vi "Log The Message.vi"(11 "Circle Message":refnum<class "Circle Message.lvclass">) -> (2 "log text":string="Draw Circle")   [LabVIEW 2019, in "Draw Messages.lvlib" / "Circle Message.lvclass"]
uses:
  Circle Message.lvclass
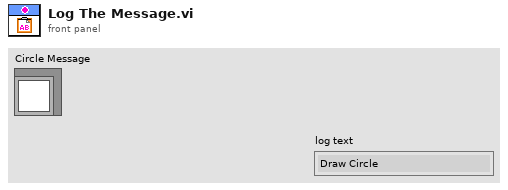
[diagram p1: front panel]
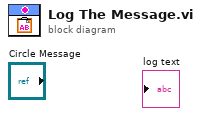
[diagram p0: block diagram]
diagram:
